vi "21.-FTP con DataSocket.vi"() -> ()   [LabVIEW 2017]
panel:
  out "Waveform Chart":dbl[][](graph)
  out "error out":errorcluster
  in  "stop":bool
  out "Waveform Graph":dbl[][](graph)
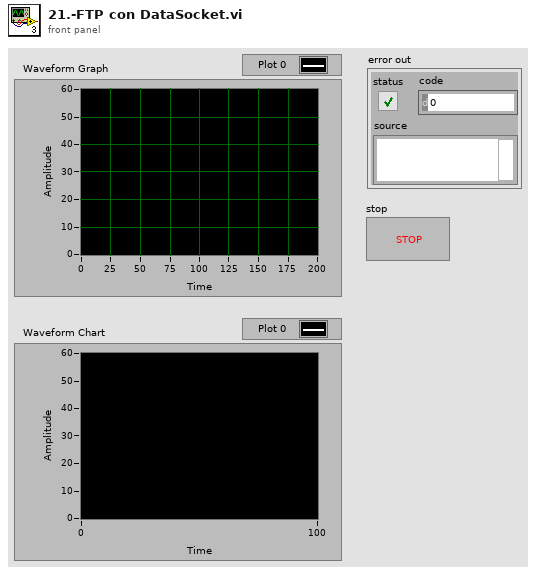
[diagram p1: front panel]
types:
  T1 = enum16{"Read", "Write", "ReadWrite", "BufferedRead", "BufferedReadWrite"}
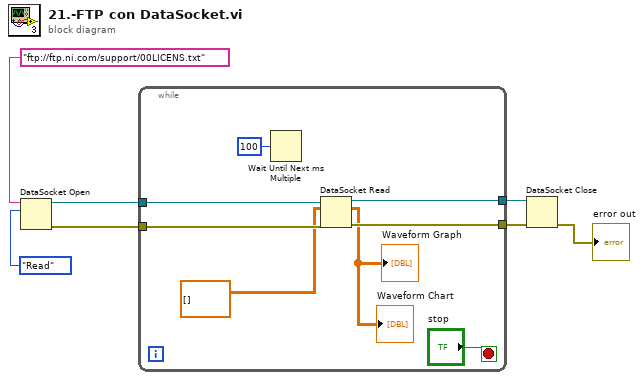
[diagram p0: block diagram]
diagram:
  n1 = DataSocket Open(10:T1."Read" ("mode"), 11:"ftp://ftp.ni.com/support/00LICENS.txt" ("URL")) -> (0:w6:errorcluster, 3:w7:refnum<k13>)  [unwired: 2 in]
  n2 = while {
    tunnel: w7 -> [w14]
    tunnel: w6 -> [w13]
    tunnel: [w12] -> w5
    tunnel: [w11] -> w4
    stop <- "stop" stop-if-true
    n3 = Wait Until Next ms Multiple(millisecond multiple=u32 100) -> ()  [unwired: 1 out]
    n4 = DataSocket Read(8:w13, 10:dbl[][] [], 11:w14) -> (0:w11:errorcluster, 2:→"Waveform Graph" →"Waveform Chart":dbl[][], 3:w12:refnum<k13>)  [unwired: 2 in, 4 out]
  }
  n5 = DataSocket Close(8:w4, 11:w5) -> (0:→"error out":errorcluster)  [unwired: 1 in, 1 out]
